vi "Add Buffer.vi"(8 "error in":errorcluster, 9 "Name":string, 10 "Buffer":refnum<data-value>, 11 "BufferMap in":refnum<data-value>) -> (0 "error out":errorcluster, 3 "BufferMap":refnum<data-value>)   [LabVIEW 2013, in "VariantBufferMap.lvclass"]
doc: "This VI writes one data element into the current location in the buffer. The location in the buffer is updated automatically."
uses:
  VariantBufferMap.lvclass
  VariantBuffer/VariantBuffer.lvclass
  VariantBufferMap.lvclass/VariantBufferMap.ctl
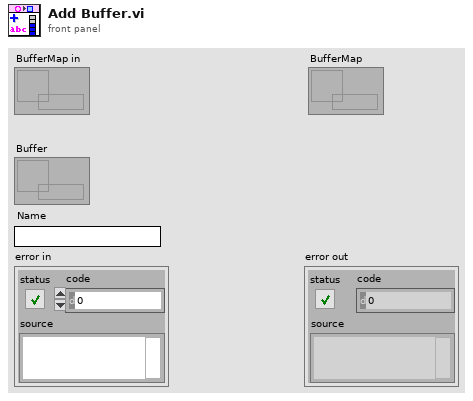
[diagram p1: front panel]
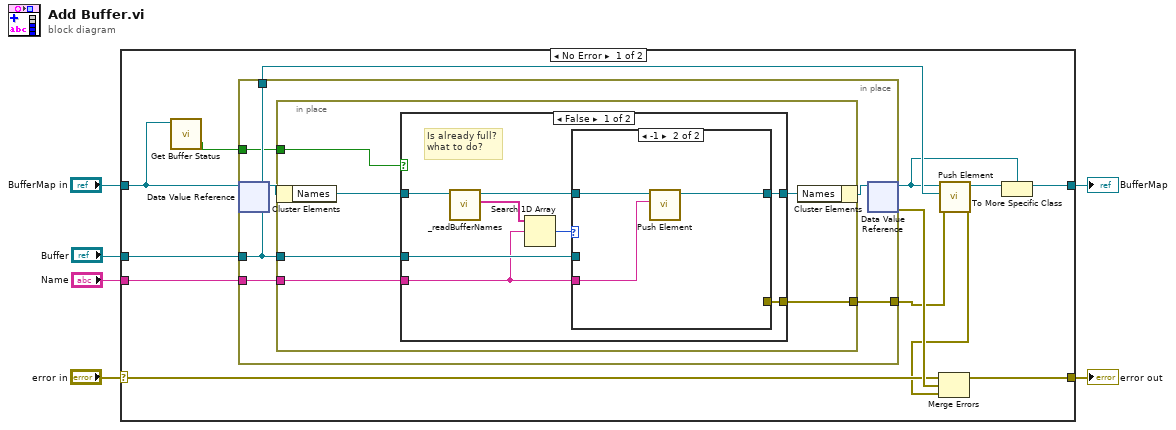
[diagram p0: block diagram]
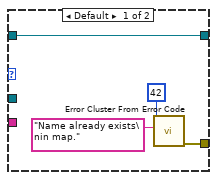
[diagram p2: hidden frame]
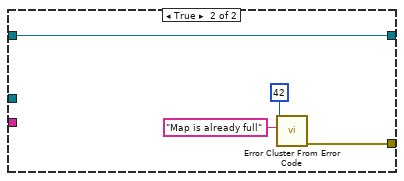
[diagram p3: hidden frame]
diagram:
  n1 = case shown="No Error" "error in" {
    selector: "error in" -> [w16 w52]
    tunnel: "BufferMap in" -> [w8 w51]
    tunnel: [w10 w51] -> w5
    tunnel: [w18 w52] -> w4
    tunnel: "Buffer" -> [w17 _]
    tunnel: "Name" -> [w15 _]
    frame No Error {
      n2 = call "Get Buffer Status.vi"("Buffer in"=w8) -> ("full"=w7:bool)  [unwired: 6 in, 4 out]
      n3 = in-place {
        in-place-border: w17 -> [w21]
        in-place-border: w15 -> [w23]
        in-place-border: [w22] -> w11
        in-place-border: [w21] -> w14
        in-place-border: w7 -> [w20]
        n4 = in-place-dvr #1(w8) -> (w25:refnum<class "VariantBufferMap.lvclass">)  [unwired: 1 out]
        n5 = in-place {
          in-place-border: w21 -> [w29]
          in-place-border: w23 -> [w28]
          in-place-border: [w27] -> w22
          in-place-border: w20 -> [w26]
          n6 = in-place-cluster #2(w25) -> ("Names"=w31:refnum<data-value>)
          n7 = case shown="False" w26 {
            tunnel: w31 -> [w39 w50]
            tunnel: [w35 w50] -> w30
            tunnel: w29 -> [w34 _]
            tunnel: w28 -> [w33 _]
            tunnel: [w32 w47] -> w27
            frame False {
              # "Is already full?\nwhat to do?"
              n8 = call "_readBufferNames.vi"("Data Value Reference in"=w39) -> ("Names"=w38:string[], "Data Value Reference out"=w36:refnum<data-value>)  [unwired: 9 in]
              n9 = Search 1D Array(1D array=w38, element=w33) -> (index of element=w37:i32)  [unwired: 1 in]
              n10 = case shown="-1" w37 {
                tunnel: w36 -> [w43 w46]
                tunnel: [w43 w45] -> w35
                tunnel: w34 -> [_ _]
                tunnel: w33 -> [_ w44]
                tunnel: [w42 _] -> w32
                frame Default {
                  n11 = call <vilib>:"Error Cluster From Error Code.vi"("error message (\"\")"="Name already exists\nin map." ("error message (\"\")"), "error code (0)"=42) -> ("error out"=w42:errorcluster)  [unwired: 7 in]
                }
                frame -1 {
                  n12 = call "Push Element.vi"("element"=w44, "Buffer in"=w46) -> ("Buffer"=w45:refnum<data-value>)  [unwired: 8 in, 1 out]
                }
              }
            }
            frame True {
              n13 = call <vilib>:"Error Cluster From Error Code.vi"("error message (\"\")"="Map is already full" ("error message (\"\")"), "error code (0)"=42) -> ("error out"=w47:errorcluster)  [unwired: 7 in]
            }
          }
          n14 = in-place-cluster #2("Names"=w30) -> (w24:refnum<class "VariantBufferMap.lvclass">)
        }
        n15 = in-place-dvr #1(w24) -> (w9:refnum<data-value>, w19:errorcluster)
      }
      n16 = call "Push Element.vi"("error in"=w11, "element"=w14, "Buffer in"=w9) -> ("error out"=w12:errorcluster, "Buffer"=w13:refnum<data-value>)  [unwired: 7 in]
      n17 = Merge Errors(w16, w19, w12) -> (w18:errorcluster)
      n18 = To More Specific Class(target class=w9, reference=w13) -> (specific class reference=w10:refnum<data-value>)  [unwired: 1 in, 1 out]
    }
    frame Error {
    }
  }
  "error out" <- w4
  "BufferMap" <- w5
